vi "CAPTH-Create Tone.vi"(0 "Freq (kHz)":dbl, 5 "runtime in":T1, 11 "error in (no error)":errorcluster) -> (4 "tone":dbl[](array[numeric]), 6 "runtime out":T1, 15 "error out":errorcluster)   [LabVIEW 2020]
uses:
  Typedefs/CAPTH-Runtime.ctl
  epl-vi-lib/PXI DAQ VIs/DAQ Engine VIs/PXI Globals.vi
panel:
  out "Waveform Graph":dbl[](graph)
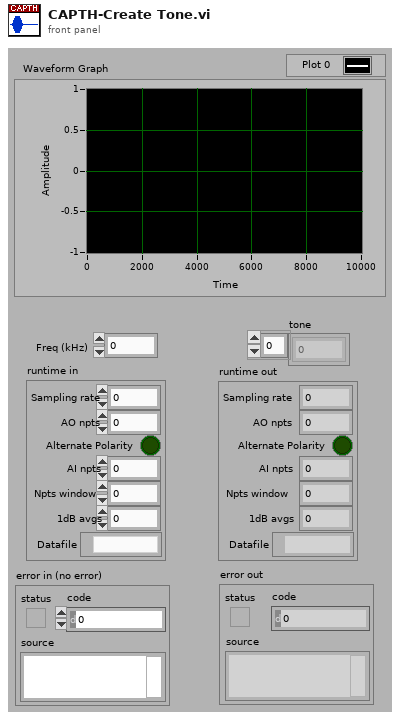
[diagram p1: front panel]
types:
  T1 = typedef "CAPTH-Runtime.ctl" = cluster{"Sampling rate":dbl, "AO npts":i32, "Alternate Polarity":bool, "AI npts":i32, "Npts window":i32, "1dB avgs":i32, "Datafile":path}
  T2 = cluster{"Active":bool, "Delay (ms)":dbl, "Width (ms)":dbl, "Ramp (ms)":dbl}
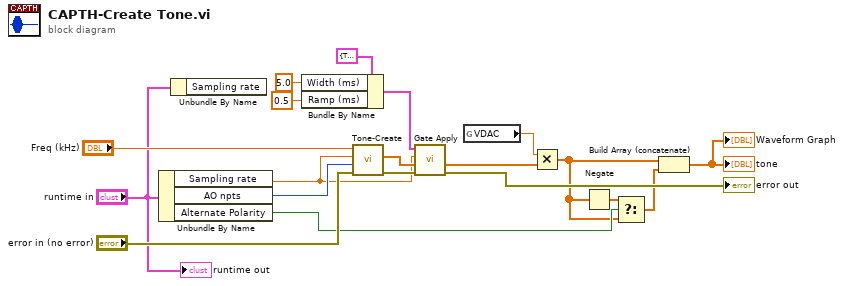
[diagram p0: block diagram]
diagram:
  n1 = Unbundle By Name("runtime in") -> ("Sampling rate"=w4:dbl, "AO npts"=w12:i32, "Alternate Polarity"=w10:bool)
  n2 = Unbundle By Name("runtime in") -> ()  [unwired: 1 out]
  n3 = Bundle By Name(cluster=T2 {"Active"=TRUE, "Delay (ms)"=0.0, "Width (ms)"=0.0, "Ramp (ms)"=0.0} ("Gate Control"), "Width (ms)"=5.0, "Ramp (ms)"=0.5) -> (w15:T2)
  n4 = call "Tone-Create.vi"("error in (no error)"="error in (no error)", "Npts"=w12, "Sampling Rate (Hz)"=w4, "Frequency (kHz)"="Freq (kHz)") -> ("error out"=w17:errorcluster, "Waveform"=w16:dbl[])  [unwired: 6 in]
  n5 = call "Gate Apply.vi"("error in (no error)"=w17, "Waveform in"=w16, "Sampling Rate (Hz)"=w4, "Gate Control"=w15) -> ("error out"=→"error out":errorcluster, "Gated waveform"=w14:dbl[])  [unwired: 6 in]
  n6 = global read "PXI Globals.vi" "VDAC"() -> (w6:dbl)
  n7 = Multiply(x=w6, y=w14) -> (x*y=w9:dbl[])
  n8 = Negate(x=w9) -> (-x=w8:dbl[])
  n9 = Select(t=w8, s=w10, f=w9) -> (s? t:f=w11:dbl[])
  n10 = Build Array (concatenate)(w9, w11) -> (→"Waveform Graph" →"tone":dbl[])
  "runtime out" <- "runtime in"
